vi "FPGA_check_dummy-channel.vi"(9 "pan-channel":u16=255) -> (1 "dummy?":bool)   [LabVIEW 2010]
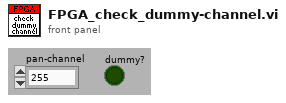
[diagram p1: front panel]
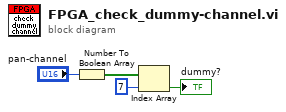
[diagram p0: block diagram]
diagram:
  n1 = Number To Boolean Array(number="pan-channel") -> (Boolean array=w3:bool[])
  n2 = Index Array(array=w3, index=7) -> (element=→"dummy?":bool)
